vi "Action.vi"(8 "error in (no error)":errorcluster, 11 "MGI_Timer.lvclass":refnum<class "MGI_Timer.lvclass">) -> (0 "error out":errorcluster, 3 "MGI_Timer.lvclass":refnum<class "MGI_Timer.lvclass">)   [LabVIEW 2016, in "MGI_Timer.lvclass"]
doc: "Authored by Derek E. Trepanier\nsupport@mooregoodideas.com\nwww.mooregoodideas.com\n\nCopyright (c) 2012, Moore Good Ideas, Inc.\n\nAll rights reserved.\n\nRedistribution and use in source and binary forms, with or without modification, are permitted provided that the following conditions are met:\n\n * Redistributions of source code must retain the above copyright notice, this list of conditions and the following disclaimer.\n * Redistributions in binary form must reproduce the above copyright notice, this list of conditions and the following disclaimer in the documentation and/or other materials provided with the distribution.\n * Neither the name of Moore Good Ideas, Inc. nor the names of its contributors may be used to endorse or promote products derived from this software without specific prior written permission.\n\nTHIS SOFTWARE IS PROVIDED BY THE COPYRIGHT HOLDERS AND CONTRIBUTORS \"AS IS\" AND ANY EXPRESS OR IMPLIED WARRANTIES, INCLUDING, BUT NOT LIMITED TO, THE IMPLIED WARRANTIES OF MERCHANTABILITY AND FITNESS FOR A PARTICULAR PURPOSE ARE DISCLAIMED. IN NO EVENT SHALL THE COPYRIGHT OWNER OR CONTRIBUTORS BE LIABLE FOR ANY DIRECT, INDIRECT, INCIDENTAL, SPECIAL, EXEMPLARY, OR CONSEQUENTIAL DAMAGES (INCLUDING, BUT NOT LIMITED TO, PROCUREMENT OF SUBSTITUTE GOODS OR SERVICES; LOSS OF USE, DATA, OR PROFITS; OR BUSINESS INTERRUPTION) HOWEVER CAUSED AND ON ANY THEORY OF LIABILITY, WHETHER IN CONTRACT, STRICT LIABILITY, OR TORT (INCLUDING NEGLIGENCE OR OTHERWISE) ARISING IN ANY WAY OUT OF THE USE OF THIS SOFTWARE, EVEN IF ADVISED OF THE POSSIBILITY OF SUCH DAMAGE."
uses:
  <userlib>/_MGI/Menu Building/Example/Plugin/Timer/MGI_Timer.lvclass
  <userlib>/_MGI/Menu Building/Example/Plugin/Timer/MGI_Timer.lvclass/MGI_Timer.ctl
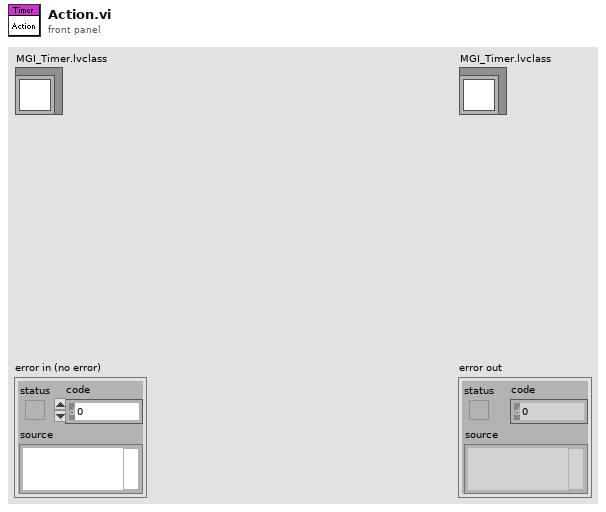
[diagram p1: front panel]
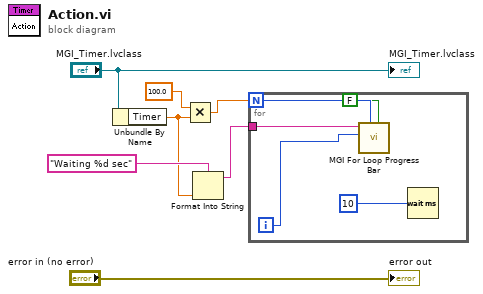
[diagram p0: block diagram]
diagram:
  n1 = Unbundle By Name("MGI_Timer.lvclass") -> ("Timer"=w2:dbl)
  n2 = Multiply(x=100.0, y=w2) -> (x*y=w5:dbl)
  n3 = Format Into String(format string="Waiting %d sec" ("Message"), w2) -> (resulting string=w1:string)  [unwired: 2 in, 1 out]
  n4 = for {
    N: w5 -> [w11]
    tunnel: w1 -> [w8]
    i -> [w12]
    n5 = call <userlib>:"MGI For Loop Progress Bar.vi"("Show Time? (T)"=FALSE, "Total Iter"=w11, "Current Iter"=w12, "Message"=w8) -> ()  [unwired: 6 in, 2 out]
    n6 = Wait (ms)(milliseconds to wait=u32 10 ("Wait Time (ms) (1000)")) -> ()  [unwired: 1 out]
  }
  "error out" <- "error in (no error)"
  "MGI_Timer.lvclass" <- "MGI_Timer.lvclass"
